vi "HasMCSRangeChanged1.vi"(0 "WFGraph Refnum":refnum<vi>) -> (1 "Selection Changed":bool, 2 "output range":cluster{"x0":dbl, "x1":dbl} {"x1" format="%.2f"; "x0" format="%.2f"})   [LabVIEW 2009]
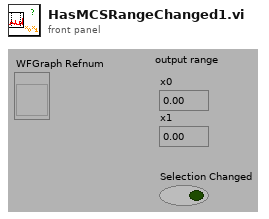
[diagram p1: front panel]
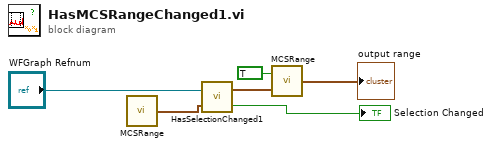
[diagram p0: block diagram]
diagram:
  n1 = call "MCSRange.vi"() -> ("output range"=w3:cluster{"x0":dbl, "x1":dbl})  [unwired: 2 in]
  n2 = call "HasSelectionChanged1.vi"("input range"=w3, "WFGraph Refnum"="WFGraph Refnum") -> ("Selection Changed"=→"Selection Changed":bool, "output range"=w5:cluster{"x0":dbl, "x1":dbl})
  n3 = call "MCSRange.vi"("input range"=w5, "set"=TRUE) -> ("output range"=→"output range":cluster{"x0":dbl, "x1":dbl})
